vi "L04.vi"() -> ()   [LabVIEW 2012]
panel:
  out "max value":i32
  out "H":i32[](array[numeric])
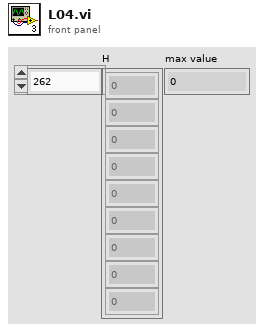
[diagram p1: front panel]
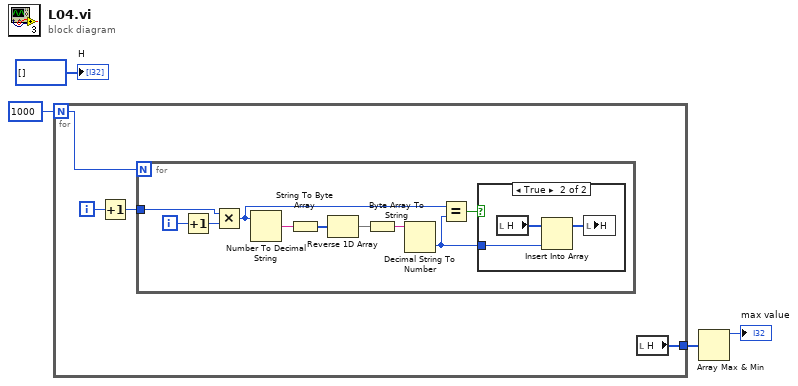
[diagram p0: block diagram]
diagram:
  n1 = for {
    N: 1000 -> [w8]
    tunnel: [w5] -> w2
    i -> [w7]
    n2 = Increment(x=w7) -> (x+1=w6:i32)
    n3 = for {
      N: w8 -> [_]
      tunnel: w6 -> [w17]
      i -> [w18]
      n4 = Increment(x=w18) -> (x+1=w9:i32)
      n5 = Multiply(x=w17, y=w9) -> (x*y=w12:i32)
      n6 = Number To Decimal String(number=w12) -> (decimal integer string=w16:string)  [unwired: 1 in]
      n7 = String To Byte Array(string=w16) -> (unsigned byte array=w15:u8[])
      n8 = Reverse 1D Array(array=w15) -> (reversed array=w14:u8[])
      n9 = Byte Array To String(unsigned byte array=w14) -> (string=w13:string)
      n10 = Decimal String To Number(string=w13) -> (number=w10:i32)  [unwired: 2 in, 1 out]
      n11 = Equal?(x=w12, y=w10) -> (x = y?=w11:bool)
      n12 = case shown="True" w11 {
        tunnel: w10 -> [_ w19]
        frame False {
        }
        frame True {
          n13 = local read "H"() -> (w21:i32[])
          n14 = Insert Into Array(array=w21, new element=w19) -> (w20:i32[])  [unwired: 1 in]
          n15 = local write "H"(w20) -> ()
        }
      }
    }
    n16 = local read "H"() -> (w5:i32[])
  }
  n17 = Array Max & Min(array=w2) -> (max value=→"max value":i32)  [unwired: 3 out]
  "H" <- i32[] []
